vi "Get Velocity.vi"   [LabVIEW 2013]
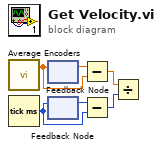
[diagram p0: block diagram]
diagram:
  n1 = call "Average Encoders.vi"() -> ("Counts"=w6:dbl)  [unwired: 1 in, 1 out]
  n2 = Tick Count (ms)() -> (millisecond timer value=w3:u32)
  n3 = feedback-in #1(w6) -> ()
  n4 = feedback #1() -> (w5:dbl)  [unwired: 1 in]
  n5 = feedback #2() -> (w4:u32)  [unwired: 1 in]
  n6 = feedback-in #2(w3) -> ()
  n7 = Subtract(x=w5, y=w6) -> (x-y=w2:dbl)
  n8 = Subtract(x=w4, y=w3) -> (x-y=w1:u32)
  n9 = Divide(x=w2, y=w1) -> ()  [unwired: 1 out]
